vi "RIOWaveformDataStore.vi"(3 "Error in":errorcluster, 4 "Experiment State":T1 {"RIO Settings"."Card Settings"."Sample Rate" format="%#_3p"; "Timing Settings"."Timing Channel Settings"."FrontPanelTime" format="%.3p"; "Timing Settings"."Timing Channel Settings"."Pulse width (s)" format="%.3p"; "Timing Settings"."Timing Channel Settings"."Delay (s)" format="%.3p"; "Digitizer Settings"."Card Settings"."Global Edge Type" items=["Rising"=10280, "Falling"=10171]; "Digitizer Settings"."Card Settings"."Sample Rate" format="%#_3p"}, 5 "Tree DVR in":refnum<data-value>) -> (0 "Error out":errorcluster)   [LabVIEW 2014]
uses:
  <vilib>/MDSplus/Classes/Tree_Class/Tree.lvclass
  Controls/ExperimentStateCluster.ctl
  Controls/DigitizerSettingsChannelSettings.ctl
  Controls/DigitizerSettingsCardSettingsArray.ctl
  Controls/DigitizerSettingsCardSettings.ctl
  Controls/TimingSettings.ctl
  Controls/TimingCardSettings.ctl
  Controls/TimingChannelSettings.ctl
  Controls/RIOSettingsExperimentStateCluster.ctl
  Controls/RIOSettingsChannelSettings.ctl
  Controls/RIOSettingsCardSettingsArray.ctl
  Controls/RIOSettingsCardSettings.ctl
  <vilib>/userdefined/High Color/nirio_resource_hc.ctl
  Controls/RIOData.ctl
  Controls/DIOChannel.ctl
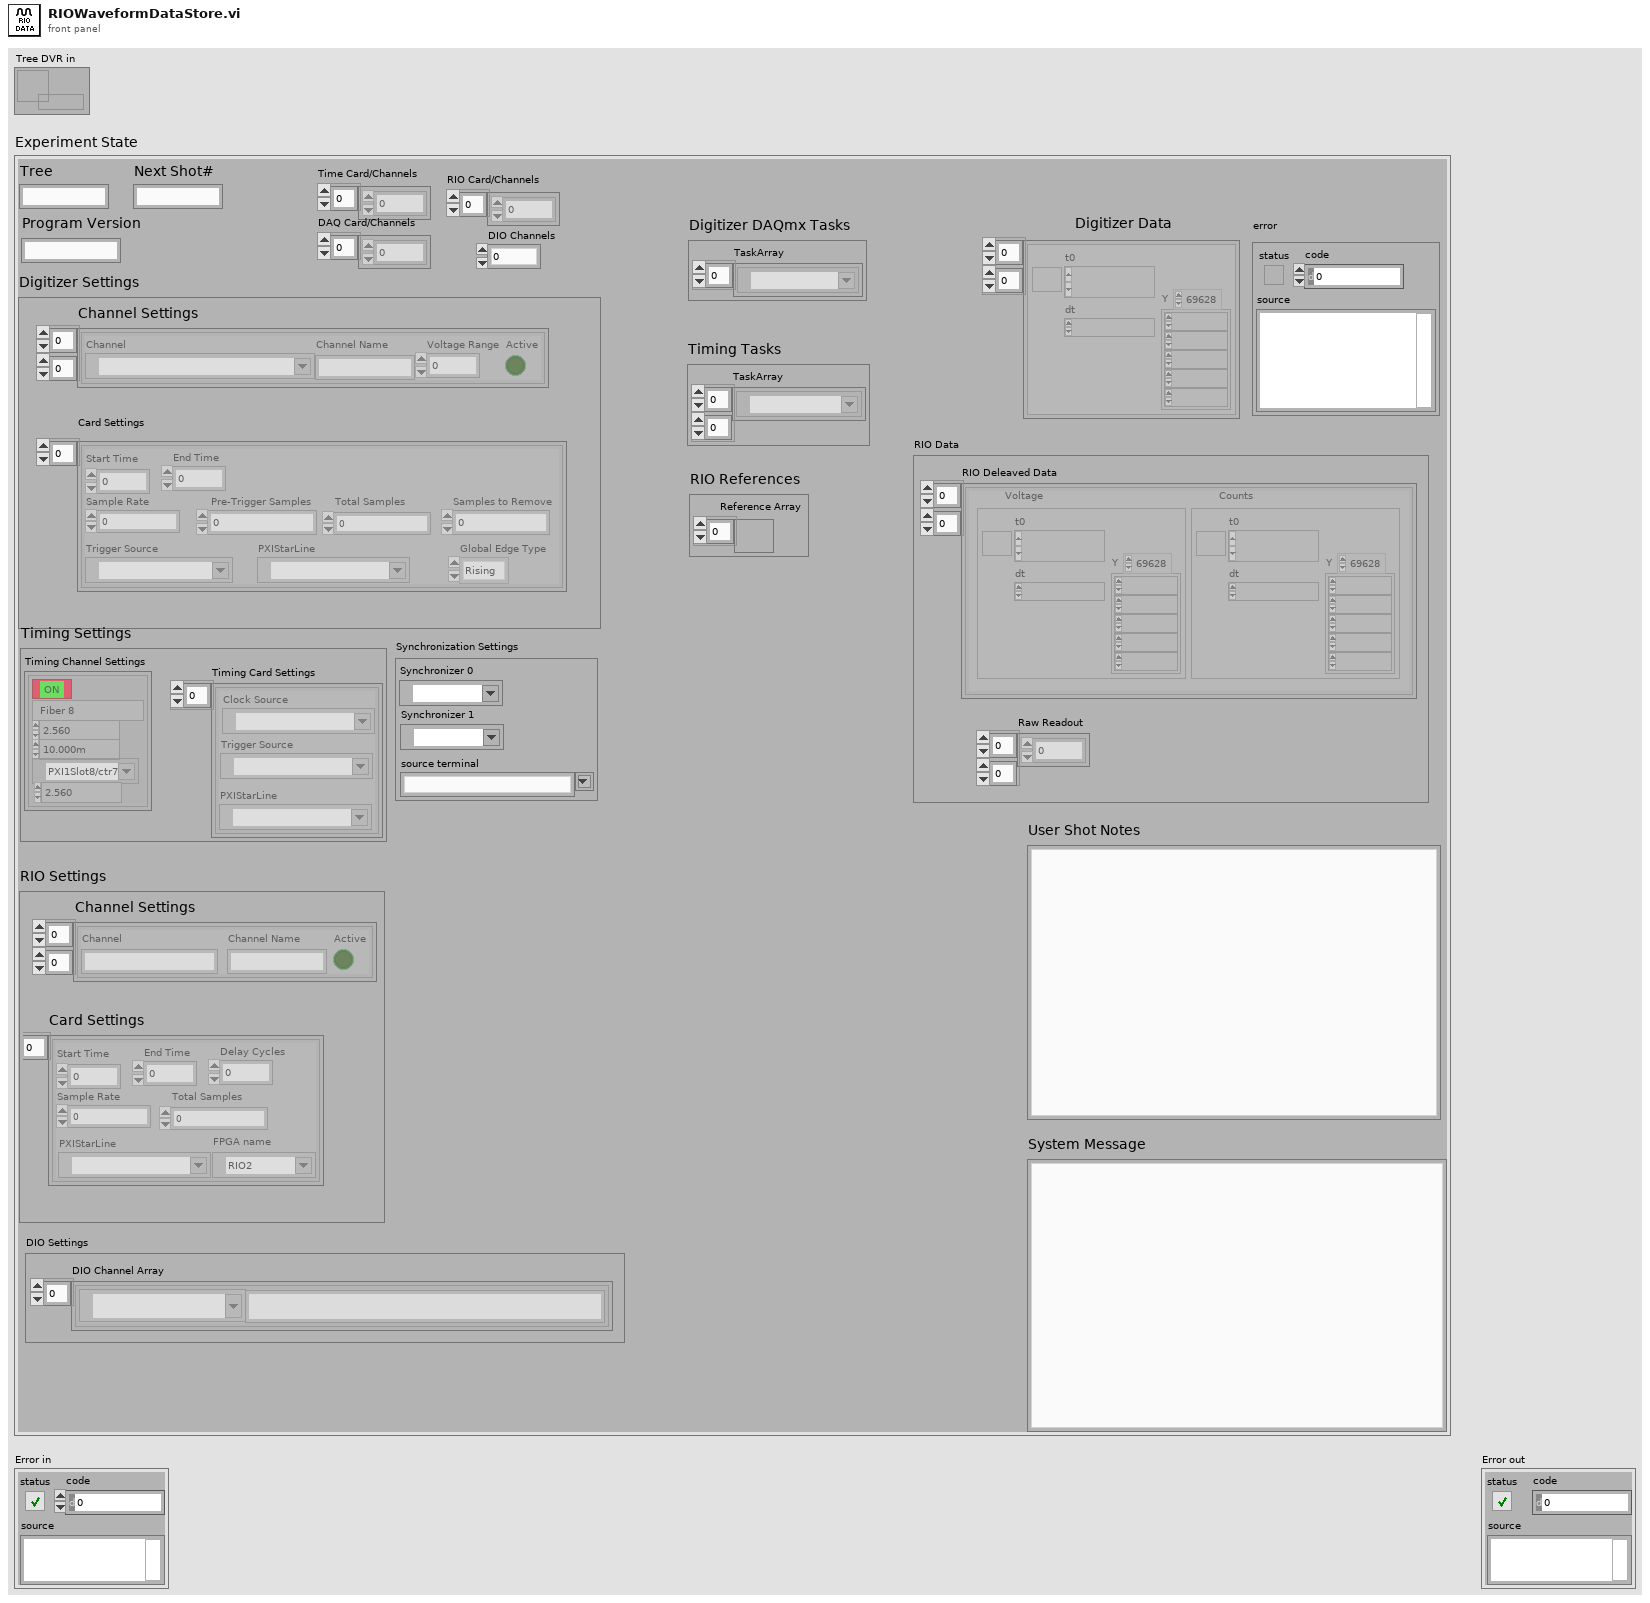
[diagram p1: front panel]
types:
  T1 = typedef "ExperimentStateCluster.ctl" = cluster{"error":errorcluster, "Digitizer DAQmx Tasks":cluster{"TaskArray":refnum<k21>[]}, "Digitizer Settings":cluster{"Channel Settings":T2[][], "Card Settings":T3}, "Synchronization Settings":cluster{"Synchronizer 0":refnum<k15>, "source terminal":string, "Synchronizer 1":refnum<k15>}, "Digitizer Data":waveform(dbl)[][], "Next Shot#":string, "System Message":string, "User Shot Notes":string, "Timing Settings":T5, "Timing Tasks":cluster{"TaskArray":refnum<k21>[][]}, "Tree":string, "Time Card/Channels":i32[], "DAQ Card/Channels":i32[], "Program Version":string, "RIO Settings":T8, "RIO References":cluster{"Reference Array":refnum<k20>[]}, "RIO Data":T13, "RIO Card/Channels":i32[], "DIO Channels":i32, "DIO Settings":cluster{"DIO Channel Array":T14[]}}
  T2 = typedef "DigitizerSettingsChannelSettings.ctl" = cluster{"Channel":tag, "Channel Name":string, "Voltage Range":dbl, "Active":bool}
  T3 = typedef "DigitizerSettingsCardSettingsArray.ctl" = T4[]
  T4 = typedef "DigitizerSettingsCardSettings.ctl" = cluster{"Start Time":dbl, "End Time":dbl, "Sample Rate":dbl, " Pre-Trigger Samples":u32, "Total Samples":i32, "Samples to Remove":u32, "Trigger Source":tag, "Global Edge Type":i32, "PXIStarLine":tag}
  T5 = typedef "TimingSettings.ctl" = cluster{"Timing Card Settings":T6[], "Timing Channel Settings":T7[][]}
  T6 = typedef "TimingCardSettings.ctl" = cluster{"Trigger Source":tag, "Clock Source":tag, "PXIStarLine":tag}
  T7 = typedef "TimingChannelSettings.ctl" = cluster{"Delay (s)":dbl, "Pulse width (s)":dbl, "Active":bool, "Channel Name":string, "counter":tag, "FrontPanelTime":dbl}
  T8 = typedef "RIOSettingsExperimentStateCluster.ctl" = cluster{"Channel Settings":T9[][], "Card Settings":T10}
  T9 = typedef "RIOSettingsChannelSettings.ctl" = cluster{"Channel Name":string, "Active":bool, "Channel":string}
  T10 = typedef "RIOSettingsCardSettingsArray.ctl" = T11[]
  T11 = typedef "RIOSettingsCardSettings.ctl" = cluster{"Start Time":dbl, "End Time":dbl, "Sample Rate":dbl, "Total Samples":u64, "PXIStarLine":tag, "Delay Cycles":u64, "FPGA name":T12}
  T12 = typedef "nirio_resource_hc.ctl" = tag
  T13 = typedef "RIOData.ctl" = cluster{"RIO Deleaved Data":cluster{"Voltage":waveform(dbl), "Counts":waveform(i16)}[][], "Raw Readout":u64[][]}
  T14 = typedef "DIOChannel.ctl" = cluster{"Channel Name":string, "NI Name":tag}
  T15 = cluster{"Voltage":waveform(dbl), "Counts":waveform(i16)}[][]
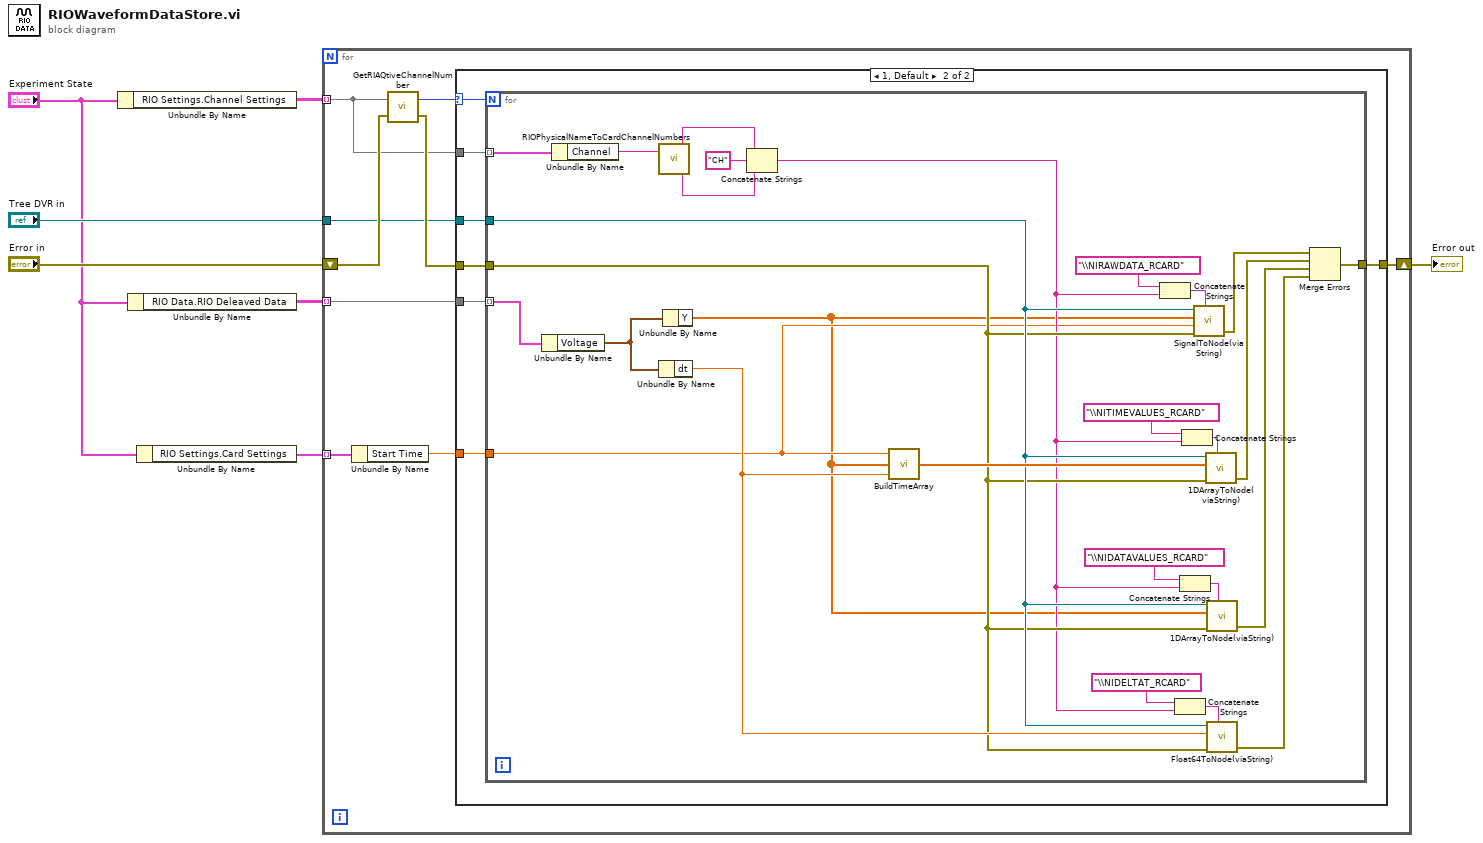
[diagram p0: block diagram]
diagram:
  n1 = Unbundle By Name("Experiment State") -> ("RIO Settings.Channel Settings"=w3:T9[][])
  n2 = Unbundle By Name("Experiment State") -> ("RIO Data.RIO Deleaved Data"=w4:T15)
  n3 = Unbundle By Name("Experiment State") -> ("RIO Settings.Card Settings"=w1:T10)
  n4 = for {
    tunnel: w4 -> [w16] mode=indexing
    shift-right: [w8] -> w6
    shift-left: "Error in" -> [w15]
    tunnel: "Tree DVR in" -> [w9]
    tunnel: w3 -> [w10] mode=indexing
    tunnel: w1 -> [w12] mode=indexing
    n5 = Unbundle By Name(w12) -> ("Start Time"=w11:dbl)
    n6 = call "GetRIAQtiveChannelNumber.vi"("error in (no error)"=w15, "Channel Settings"=w10) -> ("error out"=w14:errorcluster, "Numeric"=w13:i16)
    n7 = case shown="1, Default" w13 {
      selector: w13 -> [_ w23]
      tunnel: w16 -> [_ w24]
      tunnel: w14 -> [w17 w20]
      tunnel: w11 -> [_ w22]
      tunnel: w10 -> [_ w21]
      tunnel: w9 -> [_ w19]
      tunnel: [w17 w18] -> w8
      frame 0 {
      }
      frame 1, Default {
        n8 = for {
          N: w23 -> [_]
          tunnel: w24 -> [w51] mode=indexing
          tunnel: w22 -> [w27]
          tunnel: w21 -> [w46] mode=indexing
          tunnel: w20 -> [w32]
          tunnel: w19 -> [w33]
          tunnel: [w40] -> w18
          n9 = Unbundle By Name(w51) -> ("Voltage"=w50:waveform(dbl))
          n10 = Unbundle By Name(w46) -> ("Channel"=w45:string)
          n11 = call "RIOPhysicalNameToCardChannelNumbers.vi"("Channel Name"=w45) -> ("Channel #"=w42:string, "Card #"=w43:string)  [unwired: 1 in]
          n12 = Unbundle By Name(w50) -> ("dt"=w34:dbl)
          n13 = Unbundle By Name(w50) -> ("Y"=w26:dbl[])
          n14 = Concatenate Strings(w43, "CH" ("string"), w42) -> (w28:string)
          n15 = call "BuildTimeArray.vi"("Time Increment (dt)"=w34, "Data Array (y-values)"=w26, "Start Time (t_o)"=w27) -> ("Time Array (x-values)"=w47:dbl[])
          n16 = Concatenate Strings("\\NIRAWDATA_RCARD" ("string"), w28) -> (w41:string)
          n17 = Concatenate Strings("\\NIDELTAT_RCARD" ("string"), w28) -> (w36:string)
          n18 = Concatenate Strings("\\NIDATAVALUES_RCARD" ("string"), w28) -> (w37:string)
          n19 = Concatenate Strings("\\NITIMEVALUES_RCARD" ("string"), w28) -> (w49:string)
          n20 = call "SignalToNode(viaString).vi"("Tree DVR in"=w33, "NodePath"=w41, "y-axis (Data Range)"=w26, "Start Time"=w27, "error in (no error)"=w32) -> ("Error Message Output"=w39:errorcluster)  [unwired: 1 in, 2 out]
          n21 = call "1DArrayToNode(viaString).vi"("Tree DVR in"=w33, "DBL Array"=w47, "error in (no error)"=w32, "NodePath"=w49) -> ("error out"=w38:errorcluster)  [unwired: 1 in, 2 out]
          n22 = call "1DArrayToNode(viaString).vi"("Tree DVR in"=w33, "DBL Array"=w26, "error in (no error)"=w32, "NodePath"=w37) -> ("error out"=w31:errorcluster)  [unwired: 1 in, 2 out]
          n23 = call "Float64ToNode(viaString).vi"("Tree DVR in"=w33, "DBL in"=w34, "error in"=w32, "NodePath"=w36) -> ("error out"=w30:errorcluster)  [unwired: 1 in, 2 out]
          n24 = Merge Errors(w39, w38, w31, w30) -> (w40:errorcluster)
        }
      }
    }
  }
  "Error out" <- w6
